vi "Active Device.vi"(10 "Address":u16 format="%04x", 11 "Memory Map in":refnum<class "Memory Map.lvclass">) -> (1 "Relative Address":u16 format="%04x", 2 "Active Device":T1=enum."None", 3 "Memory Map out":refnum<class "Memory Map.lvclass">)   [LabVIEW 2021, in "Memory Map.lvclass"]
uses:
  Memory Map.lvclass
  Active Device.ctl
  Memory Map.lvclass/Memory Map.ctl
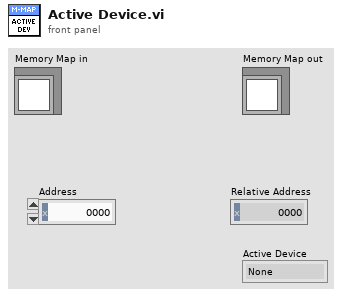
[diagram p1: front panel]
types:
  T1 = typedef "Memory Map.lvclass/Active Device.ctl" = enum16{"Error", "None", "RAM", "EEPROM", "VIA"}
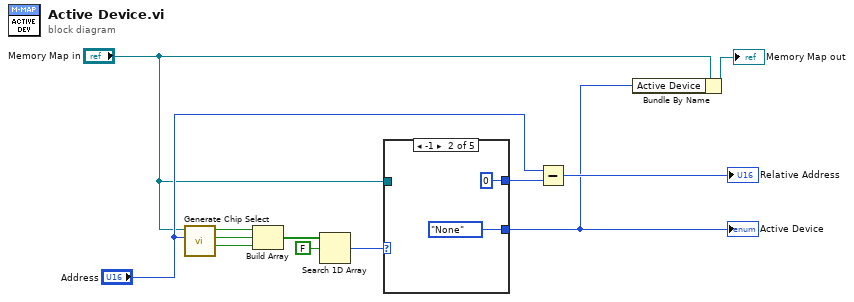
[diagram p0: block diagram]
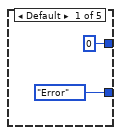
[diagram p2: hidden frame]
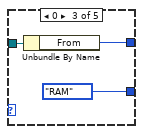
[diagram p3: hidden frame]
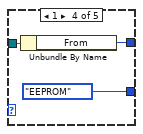
[diagram p4: hidden frame]
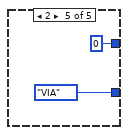
[diagram p5: hidden frame]
diagram:
  n1 = call "Generate Chip Select.vi"("Address"="Address", "Memory Map in"="Memory Map in") -> ("VIA /CS"=w7:bool, "EEPROM /CS"=w8:bool, "RAM /CS"=w12:bool)  [unwired: 7 in]
  n2 = Build Array(w12, w8, w7) -> (w11:bool[])
  n3 = Search 1D Array(1D array=w11, element=FALSE) -> (index of element=w9:i32)  [unwired: 1 in]
  n4 = case shown="-1" w9 {
    tunnel: [Active_Device."Error" ("Active Device") Active_Device."None" ("Active Device") Active_Device."RAM" ("Active Device") Active_Device."EEPROM" ("Active Device") Active_Device."VIA" ("Active Device")] -> w1
    tunnel: "Memory Map in" -> [_ _ w18 w21 _]
    tunnel: [u16 0 ("From") u16 0 ("From") w17 w20 u16 0 ("From")] -> w5
    frame Default {
    }
    frame -1 {
    }
    frame 0 {
      n5 = Unbundle By Name(w18) -> ("From"=w17:u16)
    }
    frame 1 {
      n6 = Unbundle By Name(w21) -> ("From"=w20:u16)
    }
    frame 2 {
    }
  }
  "Active Device" <- w1
  n7 = Subtract(x="Address", y=w5) -> (x-y=→"Relative Address":u16)
  n8 = Bundle By Name(cluster="Memory Map in", "Active Device"=w1) -> (→"Memory Map out":refnum<class "Memory Map.lvclass">)
